vi "Make plots.vi"(0 "Data in":T1, 1 "init":bool, 2 "reset phase":bool, 3 "nchan":i32, 5 "dt":dbl=1.0, 9 "start time":timestamp, 12 "threshold":dbl=0.1, 14 "output delay":dbl) -> (4 "plot data":waveform(dbl)[](array[waveform]), 10 "Sweep data":cluster{cluster{dbl, dbl}[]}[](array[cluster]), 15 "PSD":cluster{"f0":dbl, "df":dbl, "magnitude":dbl[]}[](array[cluster]) {"magnitude" format="%.2p"; "f0" format="%.2p"; "df" format="%.2p"})   [LabVIEW 2012]
uses:
  Data.ctl
  Treatment.ctl
  Treatment type.ctl
  <vilib>/Analysis/3filter.llb/Filter Passband Type.ctl
  <vilib>/measure/maspectr.llb/Power Spectrum and PSD Export Mode.ctl
  <vilib>/measure/maspectr.llb/FFT Power Spectrum and PSD for N Chan.vi
  <vilib>/Analysis/NI_AALPro.lvlib
  <vilib>/measure/NI_MAPro.lvlib
  <vilib>/Analysis/NI_AALBase.lvlib
panel:
  out "Data out":T1
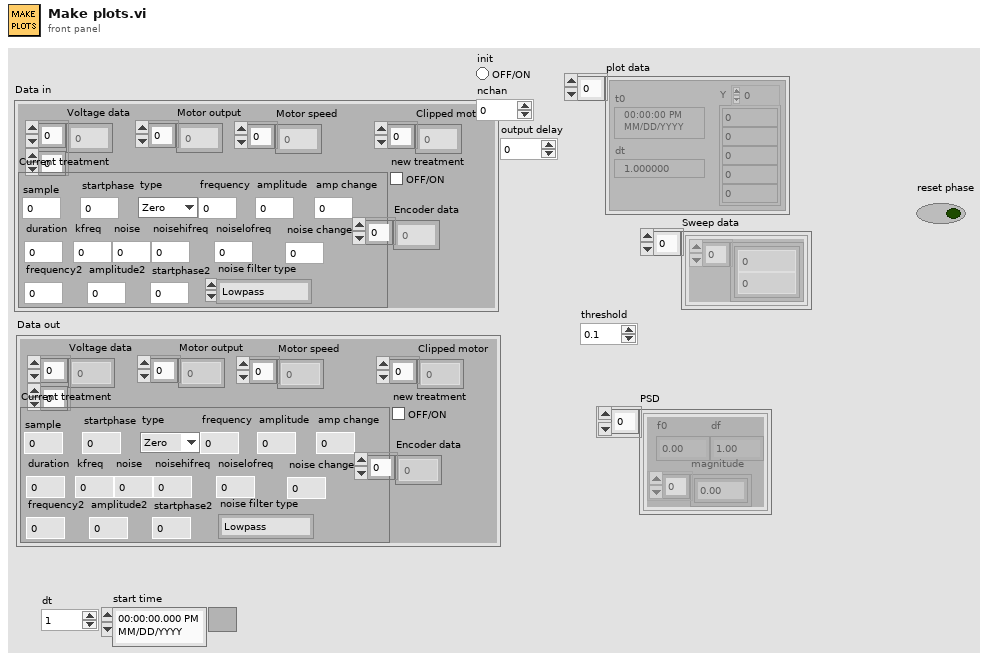
[diagram p1: front panel]
types:
  T1 = typedef "Data.ctl" = cluster{"Voltage data":dbl[][], "Encoder data":dbl[], "Motor output":dbl[], "Current treatment":T2, "Motor speed":dbl[], "Clipped motor":dbl[], "new treatment":bool}
  T2 = typedef "Treatment.ctl" = cluster{"sample":dbl, "startphase":dbl, "type":T3, "frequency":dbl, "amplitude":dbl, "noise":dbl, "duration":dbl, "kfreq":dbl, "noisehifreq":dbl, "frequency2":dbl, "amplitude2":dbl, "startphase2":dbl, "noise filter type":T4, "noiselofreq":dbl, "amp change":dbl, "noise change":dbl}
  T3 = typedef "Treatment type.ctl" = enum16{"Zero", "Sine", "Frequency sweep", "Two frequency"}
  T4 = typedef "NI_AALBase.lvlib/Filter Passband Type.ctl" = enum32{"Lowpass", "Highpass", "Bandpass", "Bandstop"}
  T5 = typedef "NI_MAPro.lvlib/Power Spectrum and PSD Export Mode.ctl" = u16
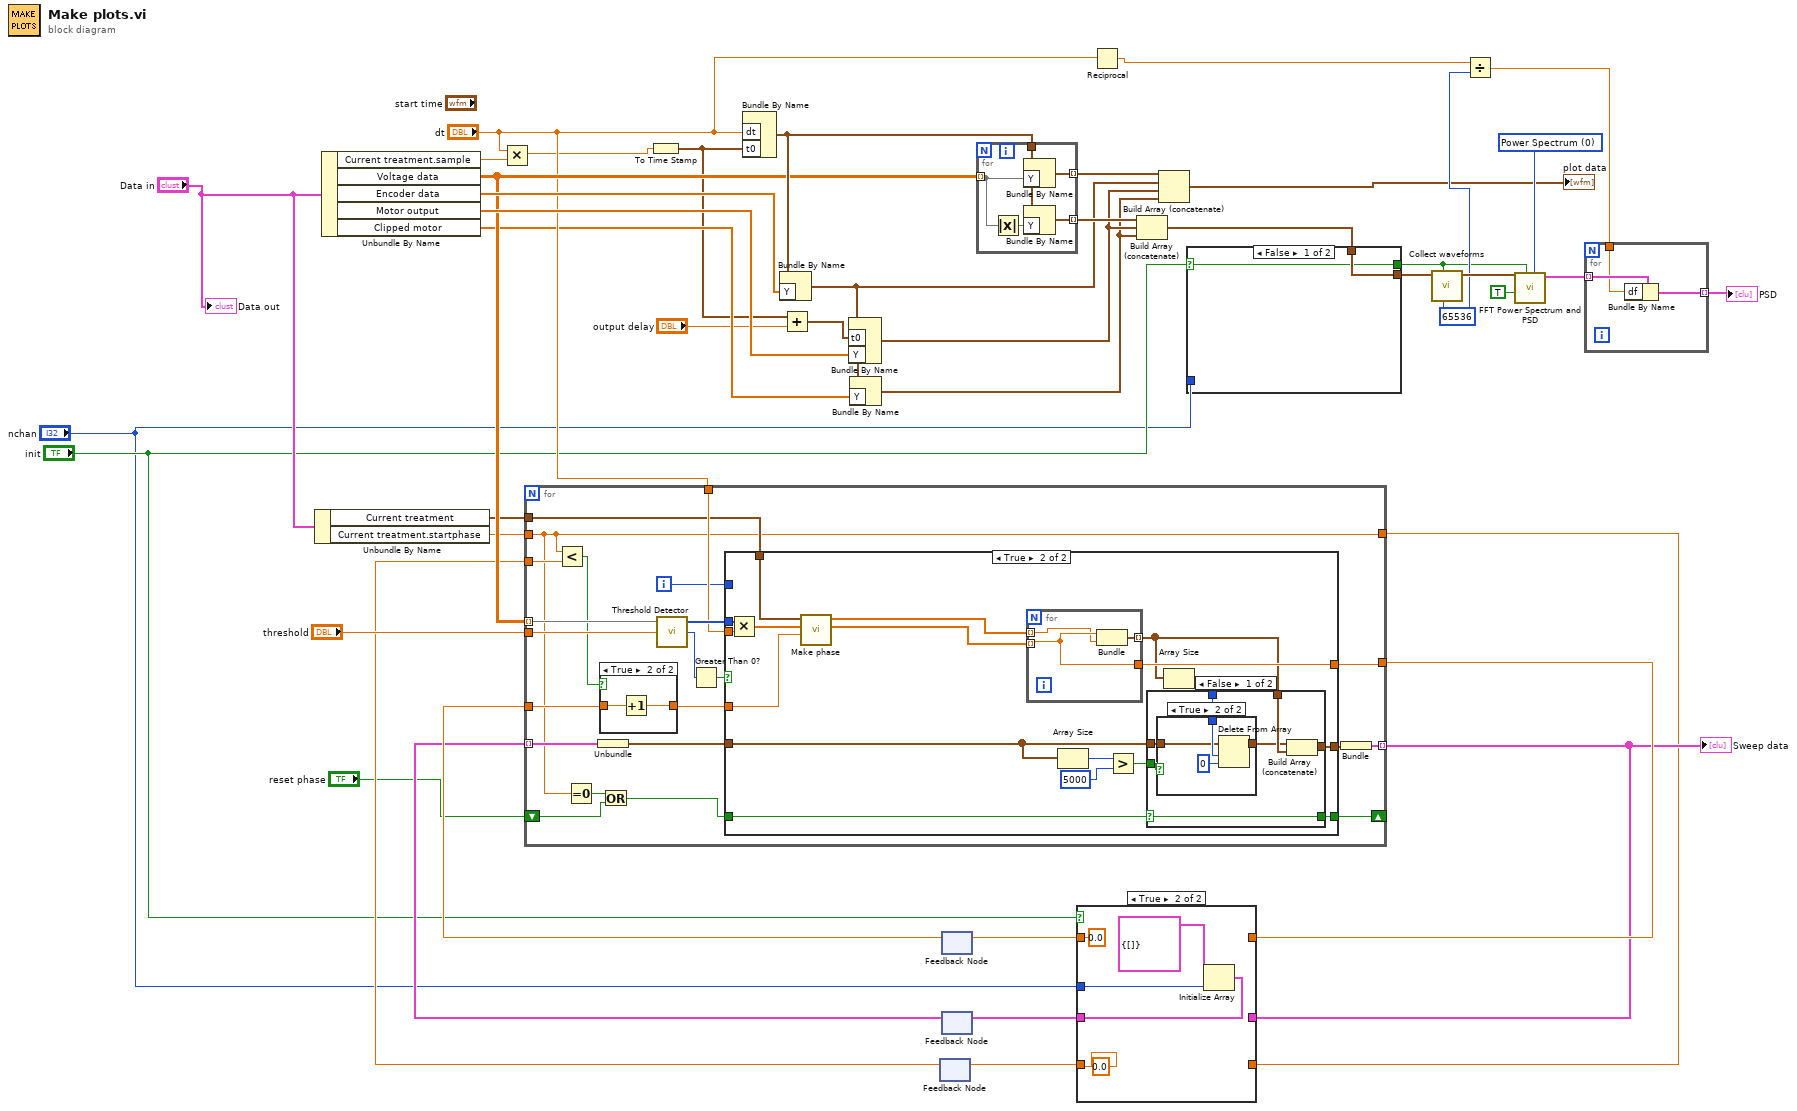
[diagram p0: block diagram]
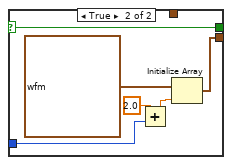
[diagram p2: hidden frame]
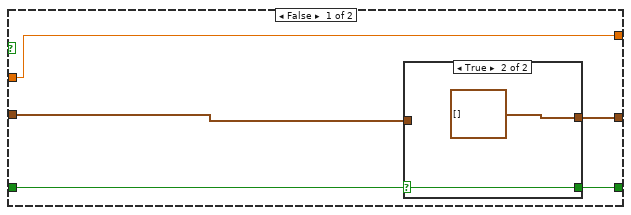
[diagram p4: hidden frame]
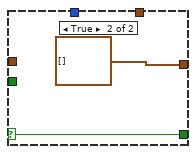
[diagram p7: hidden frame]
diagram:
  w25 = T5 0 items=["Power Spectrum", "Power Spectral Density"] ("export mode")
  w19 = 65536 ("max len")
  n1 = Unbundle By Name("Data in") -> ("Current treatment"=w36:T2, "Current treatment.startphase"=w13:dbl)
  n2 = Unbundle By Name("Data in") -> ("Current treatment.sample"=w44:dbl, "Voltage data"=w39:dbl[][], "Encoder data"=w43:dbl[], "Motor output"=w41:dbl[], "Clipped motor"=w9:dbl[])
  n3 = Multiply(x="dt", y=w44) -> (x*y=w2:dbl)
  n4 = To Time Stamp(1:w2) -> (0:w3:timestamp)
  n5 = Bundle By Name("dt"="dt", "t0"=w3) -> (w42:waveform(dbl))  [unwired: 1 in]
  n6 = Bundle By Name(cluster=w42, "Y"=w43) -> (w4:waveform(dbl))
  n7 = Add(x=w3, y="output delay") -> (x+y=w5:timestamp)
  n8 = Bundle By Name(cluster=w4, "t0"=w5, "Y"=w41) -> (w8:waveform(dbl))
  n9 = Bundle By Name(cluster=w8, "Y"=w9) -> (w7:waveform(dbl))
  n10 = feedback #1() -> (w27:dbl)  [unwired: 1 in]
  n11 = feedback #2() -> (w31:dbl)  [unwired: 1 in]
  n12 = feedback #3() -> (w30:cluster{cluster{dbl, dbl}[]}[])  [unwired: 1 in]
  n13 = for {
    tunnel: w39 -> [w66] mode=indexing
    tunnel: "threshold" -> [w65]
    tunnel: "dt" -> [w63]
    tunnel: w36 -> [w62]
    tunnel: w13 -> [w48]
    tunnel: [w61] -> w35
    tunnel: w31 -> [w55]
    tunnel: w30 -> [w60] mode=indexing
    tunnel: [w58] -> w33 mode=indexing
    tunnel: [w48] -> w29
    tunnel: w27 -> [w56]
    shift-right: [w49] -> _
    shift-left: "reset phase" -> [w46]
    i -> [w50]
    n14 = Less?(x=w48, y=w56) -> (x < y?=w54:bool)
    n15 = Equal To 0?(x=w48) -> (x = 0?=w47:bool)
    n16 = Unbundle(w60) -> (w57:cluster{dbl, dbl}[])
    n17 = case shown="True" w54 {
      tunnel: w55 -> [w110 w112]
      tunnel: [w110 w111] -> w53
      frame False {
      }
      frame True {
        n18 = Increment(x=w112) -> (x+1=w111:dbl)
      }
    }
    n19 = Or(x=w47, y=w46) -> (x .or. y?=w45:bool)
    n20 = call <vilib>:"Threshold Detector.vi"("threshold"=w65, "X"=w66) -> ("count"=w52:i32, "Indices"=w64:i32[])  [unwired: 1 in, 1 out]
    n21 = Greater Than 0?(x=w52) -> (x > 0?=w51:bool)
    n22 = case shown="True" w51 {
      tunnel: w64 -> [_ w92]
      tunnel: w63 -> [_ w91]
      tunnel: w62 -> [_ w84]
      tunnel: [w71 w90] -> w61
      tunnel: [w68 w77] -> w59
      tunnel: w57 -> [w69 w88]
      tunnel: w53 -> [w71 w82]
      tunnel: w45 -> [w70 w79]
      tunnel: w50 -> [_ _]
      tunnel: [w67 w76] -> w49
      frame False {
        n23 = case shown="True" w70 {
          selector: w70 -> [w73 w74]
          tunnel: [w72 cluster{dbl, dbl}[] []] -> w68
          tunnel: [w73 w74] -> w67
          tunnel: w69 -> [w72 _]
          frame False {
          }
          frame True {
          }
        }
      }
      frame True {
        n24 = Multiply(x=w92, y=w91) -> (x*y=w83:dbl[])
        n25 = call "Make phase.vi"("previous cycle"=w82, "Time"=w83, "Current treatment"=w84) -> ("cycle"=w81:dbl[], "phase"=w80:dbl[])  [unwired: 7 in]
        n26 = for {
          tunnel: w80 -> [w107] mode=indexing
          tunnel: w81 -> [w108] mode=indexing
          tunnel: [w109] -> w78 mode=indexing
          tunnel: [w108] -> w90
          n27 = Bundle(w108, w107) -> (w109:cluster{dbl, dbl})  [unwired: 1 in]
        }
        n28 = Array Size(array=w88) -> (size(s)=w87:i32)
        n29 = Greater?(x=w87, y=5000) -> (0:w85:bool)
        n30 = Array Size(array=w78) -> (size(s)=w89:i32)
        n31 = case shown="False" w79 {
          selector: w79 -> [w93 w105]
          tunnel: w89 -> [w99 _]
          tunnel: [w94 cluster{dbl, dbl}[] []] -> w77
          tunnel: w88 -> [w98 _]
          tunnel: w85 -> [w97 _]
          tunnel: w78 -> [w96 _]
          tunnel: [w93 w105] -> w76
          frame False {
            n32 = case shown="True" w97 {
              tunnel: w99 -> [_ w104]
              tunnel: [w100 w102] -> w95
              tunnel: w98 -> [w100 w101]
              frame False {
              }
              frame True {
                n33 = Delete From Array(array=w101, length=w104, index=0) -> (array with subset deleted=w102:cluster{dbl, dbl}[])  [unwired: 1 out]
              }
            }
            n34 = Build Array (concatenate)(w95, w96) -> (w94:cluster{dbl, dbl}[])
          }
          frame True {
          }
        }
      }
    }
    n35 = Bundle(w59) -> (w58:cluster{cluster{dbl, dbl}[]})  [unwired: 1 in]
  }
  "Sweep data" <- w33
  n36 = for {
    tunnel: w39 -> [w115] mode=indexing
    tunnel: w42 -> [w116]
    tunnel: [w117] -> w40 mode=indexing
    tunnel: [w113] -> w11 mode=indexing
    n37 = Absolute Value(x=w115) -> (abs(x)=w114:dbl[])
    n38 = Bundle By Name(cluster=w116, "Y"=w115) -> (w117:waveform(dbl))
    n39 = Bundle By Name(cluster=w116, "Y"=w114) -> (w113:waveform(dbl))
  }
  n40 = case shown="True" "init" {
    tunnel: w35 -> [w120 _]
    tunnel: [w120 0.0] -> w34
    tunnel: w33 -> [w119 _]
    tunnel: [w119 w123] -> w32
    tunnel: [w118 0.0] -> w28
    tunnel: w29 -> [w118 _]
    tunnel: "nchan" -> [_ w121]
    frame False {
    }
    frame True {
      n41 = Initialize Array(cluster{cluster{dbl, dbl}[]} {[]}, w121) -> (w123:cluster{cluster{dbl, dbl}[]}[])
    }
  }
  n42 = feedback-in #1(w28) -> ()
  n43 = feedback-in #2(w34) -> ()
  n44 = feedback-in #3(w32) -> ()
  n45 = Reciprocal(x="dt") -> (1/x=w18:dbl)
  n46 = Build Array (concatenate)(w11, w8, w7) -> (w10:waveform(dbl)[])
  n47 = Build Array (concatenate)(w40, w4, w8, w7) -> (→"plot data":waveform(dbl)[])
  n48 = case shown="False" "init" {
    selector: "init" -> [w126 w128]
    tunnel: "nchan" -> [_ w131]
    tunnel: w10 -> [w127 _]
    tunnel: [w127 w129] -> w15
    tunnel: [w126 w128] -> w14
    frame False {
    }
    frame True {
      n49 = Add(x=2.0, y=w131) -> (x+y=w130:dbl)
      n50 = Initialize Array(waveform(dbl) {"t0"=timestamp(0 s since 1904-01-01), "dt"=1.0, "Y"=[]} ("output waveform"), w130) -> (w129:waveform(dbl)[])
    }
  }
  n51 = call "Collect waveforms.vi"("max len"=w19, "init"=w14, "waveforms"=w15) -> ("waveforms out"=w26:waveform(dbl)[])  [unwired: 8 in]
  n52 = Divide(x=w18, y=w19) -> (x/y=w20:dbl)
  n53 = call-poly <vilib>:"FFT Power Spectrum and PSD.vi"("export mode"=w25, "restart averaging (F)"=w14, "dB On (F)"=TRUE, "time signals"=w26) -> ("Power Spectrum / PSD"=w23:cluster{"f0":dbl, "df":dbl, "magnitude":dbl[]}[])  [unwired: 4 in, 3 out]
  n54 = for {
    tunnel: w23 -> [w136] mode=indexing
    tunnel: w20 -> [w135]
    tunnel: [w134] -> w21 mode=indexing
    n55 = Bundle By Name(cluster=w136, "df"=w135) -> (w134:cluster{"f0":dbl, "df":dbl, "magnitude":dbl[]})
  }
  "PSD" <- w21
  "Data out" <- "Data in"
